vi "read_params.vi"(8 "error in (no error)":errorcluster, 11 "GradientBoostingClassifier in":refnum<class "GradientBoostingClassifier.lvclass">) -> (0 "error out":errorcluster, 2 "params":T1={"loss"="deviance", "learning_rate"=0.1, "n_estimators"=100.0, "subsample"=1.00000001, "criterion"="friedman_mse", "min_samples_split"=2.0, "min_samples_leaf"=1.0, "min_weight_fraction_leaf"=0.0, "max_depth"={"max_depth_type"="int", "max_depth_int"=3.0}, "min_impurity_decrease"=0.0, "init"="None", "random_state"=0.0, "max_features"={"max_features_type"="None", "max_features_float"=1.0, "max_features_int"=0.0}, "verbose"=0.0, "max_leaf_nodes"={"max_leaf_nodes_type"="None", "max_leaf_nodes_int"=0.0}, "warm_start"=FALSE, "validation_fraction"=0.1, "n_iter_no_change"={"n_iter_no_change_type"="None", "n_iter_no_change_int"=0.0}, "tol"=0.0001, "ccp_alpha"=0.0}, 3 "GradientBoostingClassifier out":refnum<class "GradientBoostingClassifier.lvclass">)   [LabVIEW 2020, in "GradientBoostingClassifier.lvclass"]
uses:
  GradientBoostingClassifier.lvclass
  Controls/gradient_boosting_classifier_params.ctl
  GradientBoostingClassifier.lvclass/GradientBoostingClassifier.ctl
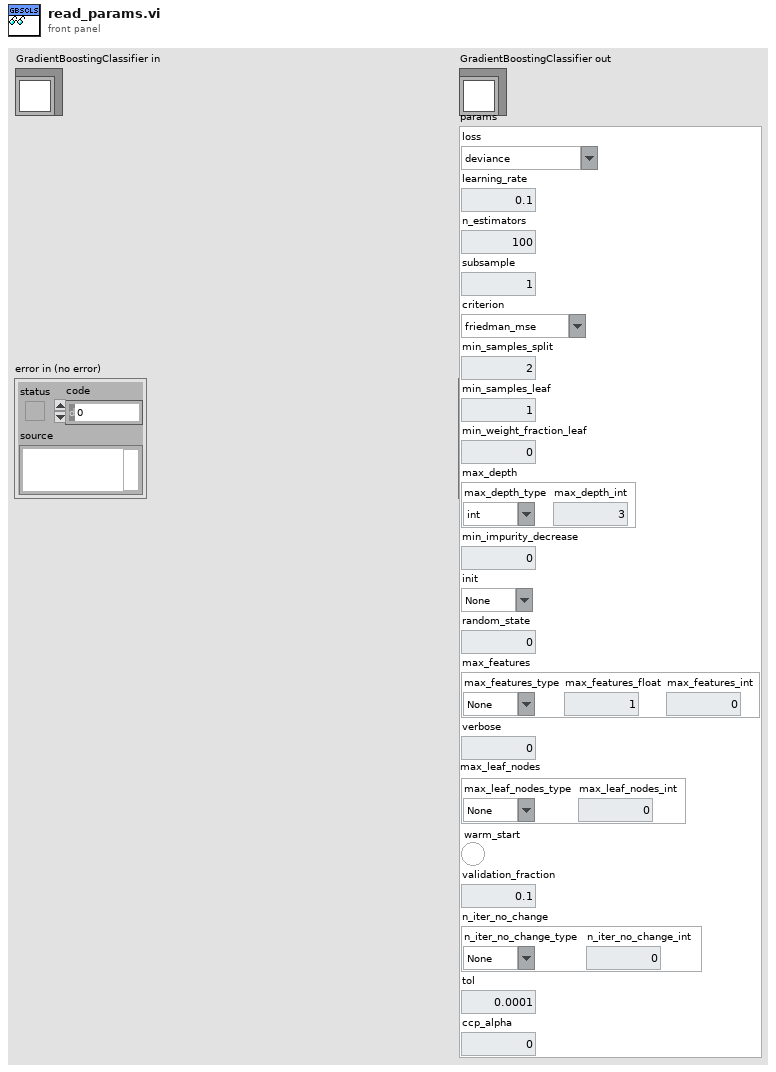
[diagram p1: front panel]
types:
  T1 = typedef "gradient_boosting_classifier_params.ctl" = cluster{"loss":string, "learning_rate":dbl, "n_estimators":dbl, "subsample":dbl, "criterion":string, "min_samples_split":dbl, "min_samples_leaf":dbl, "min_weight_fraction_leaf":dbl, "max_depth":cluster{"max_depth_type":string, "max_depth_int":dbl}, "min_impurity_decrease":dbl, "init":string, "random_state":dbl, "max_features":cluster{"max_features_type":string, "max_features_float":dbl, "max_features_int":dbl}, "verbose":dbl, "max_leaf_nodes":cluster{"max_leaf_nodes_type":string, "max_leaf_nodes_int":dbl}, "warm_start":bool, "validation_fraction":dbl, "n_iter_no_change":cluster{"n_iter_no_change_type":string, "n_iter_no_change_int":dbl}, "tol":dbl, "ccp_alpha":dbl}
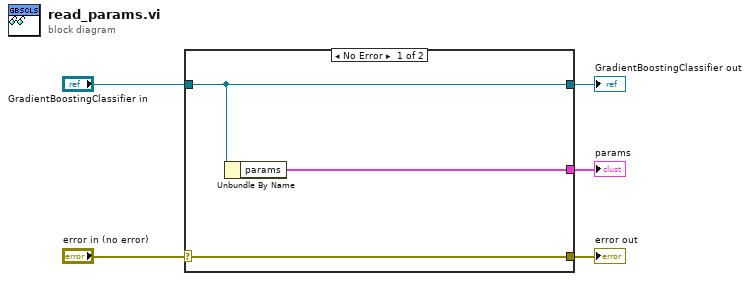
[diagram p0: block diagram]
diagram:
  n1 = case shown="No Error" "error in (no error)" {
    selector: "error in (no error)" -> [w8 w9]
    tunnel: [w8 w9] -> w4
    tunnel: [w7 w10] -> w2
    tunnel: "GradientBoostingClassifier in" -> [w7 w10]
    tunnel: [w6 _] -> w1
    frame No Error {
      n2 = Unbundle By Name(w7) -> ("params"=w6:T1)
    }
    frame Error {
    }
  }
  "error out" <- w4
  "GradientBoostingClassifier out" <- w2
  "params" <- w1
